vi "IsLeapYear.vi"(4 "Year":i32) -> (1 "Is leap year?":bool)   [LabVIEW 2017, in "GPTiming.lvlib"]
doc: "Calculates if <B>Year</B> is a leap year.\n\nSteen Schmidt\nGPower\n14/4 2016"
uses:
  GPTiming.lvlib
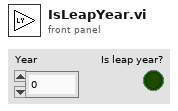
[diagram p1: front panel]
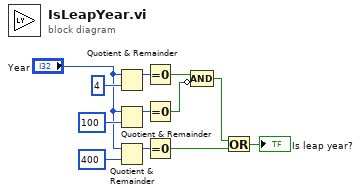
[diagram p0: block diagram]
diagram:
  n1 = Quotient & Remainder(x="Year", y=4) -> (x-y*floor(x/y)=w11:i32)  [unwired: 1 out]
  n2 = Quotient & Remainder(x="Year", y=100) -> (x-y*floor(x/y)=w10:i32)  [unwired: 1 out]
  n3 = Quotient & Remainder(x="Year", y=400) -> (x-y*floor(x/y)=w7:i32)  [unwired: 1 out]
  n4 = Equal To 0?(x=w11) -> (x = 0?=w5:bool)
  n5 = Equal To 0?(x=w10) -> (x = 0?=w4:bool)
  n6 = Equal To 0?(x=w7) -> (x = 0?=w3:bool)
  n7 = Compound Arithmetic op=AND(w5, invert w4) -> (w2:bool)
  n8 = Or(x=w2, y=w3) -> (x .or. y?=→"Is leap year?":bool)
